vi "Close first FITS Reference.vi"(8 "error in (no error)":errorcluster, 11 "Save Image in":refnum<class "Save Image.lvclass">) -> (0 "error out":errorcluster, 3 "Save Image out":refnum<class "Save Image.lvclass">)   [LabVIEW 2018, in "Save Image.lvclass"]
uses:
  Save Image.lvclass
  <userlib>/gfitsio/gfitsio.lvlib
  Simulated_Header/Simulated_Header.lvclass
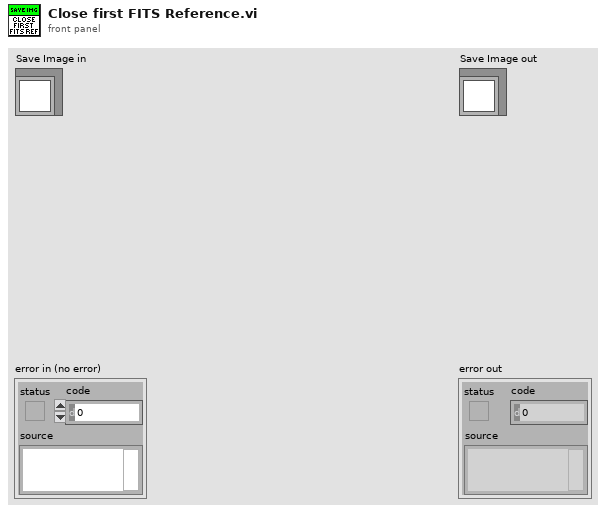
[diagram p1: front panel]
types:
  T1 = typedef "gfitsio.lvlib/gfitsio-refnum.ctl" = refnum<k1>
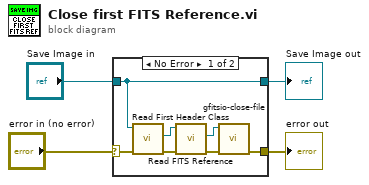
[diagram p0: block diagram]
diagram:
  n1 = case shown="No Error" "error in (no error)" {
    selector: "error in (no error)" -> [w5 w13]
    tunnel: [w11 w13] -> w3
    tunnel: [w8 w12] -> w1
    tunnel: "Save Image in" -> [w8 w12]
    frame No Error {
      n2 = call "Read First Header Class.vi"("error in (no error)"=w5, "Save Image in"=w8) -> ("error out"=w6:errorcluster, "Simulated_Header.lvclass"=w7:refnum<class "Simulated_Header.lvclass">)  [unwired: 7 in, 1 out]
      n3 = call "Read FITS Reference.vi"("error in (no error)"=w6, "Simulated_Header in"=w7) -> ("error out"=w10:errorcluster, "gfits refnum"=w9:T1)  [unwired: 7 in, 1 out]
      n4 = call <userlib>:"gfitsio-close-file.vi"("error in (no error)"=w10, "gfits refnum"=w9) -> ("error out"=w11:errorcluster)  [unwired: 8 in, 1 out]
    }
    frame Error {
    }
  }
  "error out" <- w3
  "Save Image out" <- w1
